vi "brewster error.vi"(10 "Error (grados)":dbl, 11 "Numeric Control":dbl) -> (2 "Índice de Refracción +error":dbl, 3 "Ángulo de Brewster +error":dbl)   [LabVIEW 2025]
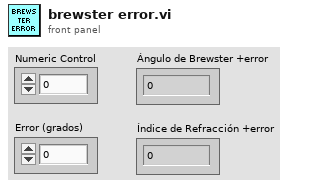
[diagram p1: front panel]
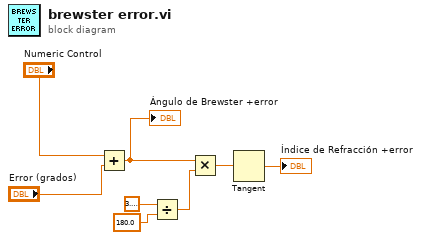
[diagram p0: block diagram]
diagram:
  n1 = Add(x="Numeric Control", y="Error (grados)") -> (x+y=w3:dbl)
  "Ángulo de Brewster +error" <- w3
  n2 = Divide(x=3.141592653589793, y=180.0) -> (x/y=w6:dbl)
  n3 = Multiply(x=w3, y=w6) -> (x*y=w7:dbl)
  n4 = Tangent(1:w7) -> (0:→"Índice de Refracción +error":dbl)
